vi "pb_select_board.vi"(8 "error in (no error)":errorcluster, 10 "board_num":i32, 11 "path in":path) -> (0 "error out":errorcluster, 3 "path out":path)   [LabVIEW 2012]
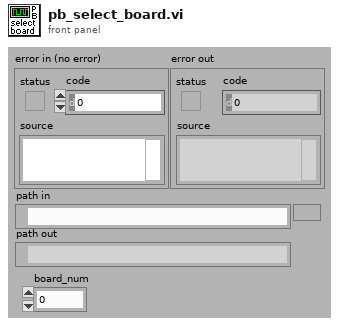
[diagram p1: front panel]
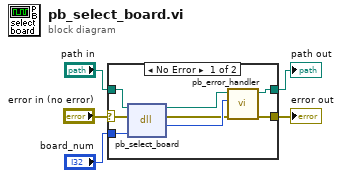
[diagram p0: block diagram]
diagram:
  n1 = case shown="No Error" "error in (no error)" {
    selector: "error in (no error)" -> [w13 w15]
    tunnel: [w7 w15] -> w4
    tunnel: "path in" -> [w11 w14]
    tunnel: [w9 w14] -> w2
    tunnel: "board_num" -> [w6 _]
    frame No Error {
      n2 = dll-call lib="C:/Program Files/SpinCore/SpinAPI/dll/spinapi.dll" fn="pb_select_board"(path in=w11, error in=w13, "board_num"=w6) -> (path out=w10:path, error out=w8:errorcluster, "return type"=w12:i32)  [unwired: 2 in]
      n3 = call "pb_error_handler.vi"("error in (no error)"=w8, "return code"=w12, "path in"=w10) -> ("error out"=w7:errorcluster, "path out"=w9:path)  [unwired: 7 out]
    }
    frame Error {
    }
  }
  "error out" <- w4
  "path out" <- w2
